vi "Binary_SpectroscopyFile-Open.vi"(8 "error in (no error)":errorcluster, 11 "Binary Spectroscopy File":path) -> (0 "error out":errorcluster, 1 "Config":T1, 2 "Number of Experiments":i32, 3 "File ref":refnum<file>, 5 "Global Attributes":string[][](table))   [LabVIEW 2021, in "Nanonis Prog Interface.lvlib"]
doc: "<b>Opens a binary (.3ds) file and reads the header.</b>\n\nIt will return the file configuration (cluster containing grid resolution, grid position & size, acquired channels etc.) and a file reference.\n\n- Nanonis Programming Interface -"
uses:
  Nanonis Prog Interface.lvlib
  Binary_SpectroscopyFile-Config.ctl
panel:
  out "file size (bytes)":i32
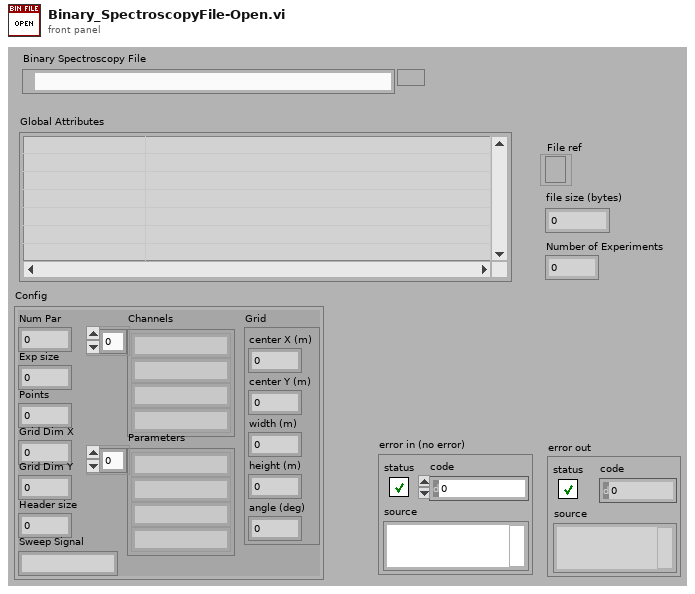
[diagram p1: front panel]
types:
  T1 = typedef "Nanonis Prog Interface.lvlib/Binary_SpectroscopyFile-Config.ctl" = cluster{"Num Par":i32, "Exp size":i32, "Points":i32, "Grid Dim X":i32, "Grid Dim Y":i32, "Header size":i32, "Channels":string[], "Parameters":string[], "Sweep Signal":string, "Grid":cluster{"center X (m)":sgl, "center Y (m)":sgl, "width (m)":sgl, "height (m)":sgl, "angle (deg)":sgl}}
  T2 = cluster{"center X":sgl, "center Y":sgl, "width":sgl, "height":sgl, "angle":sgl}
  T3 = cluster{"[0]":sgl, "[1]":sgl, "[2]":sgl, "[3]":sgl, "[4]":sgl}
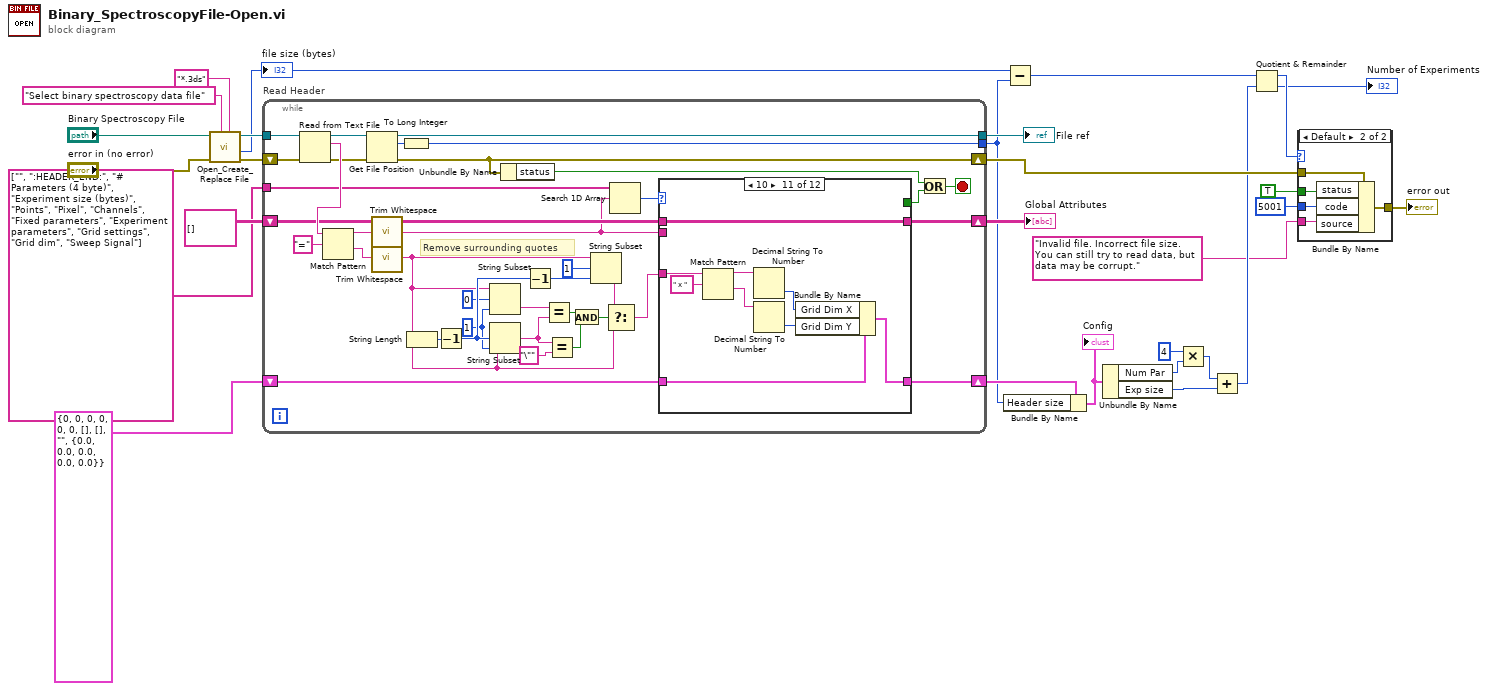
[diagram p0: block diagram]
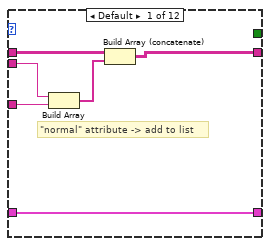
[diagram p3: hidden frame]
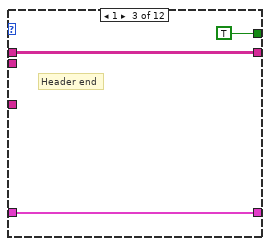
[diagram p5: hidden frame]
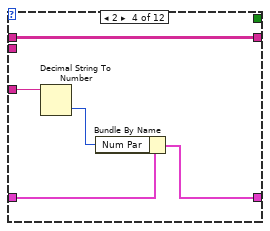
[diagram p6: hidden frame]
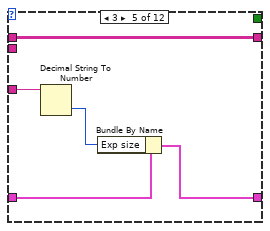
[diagram p7: hidden frame]
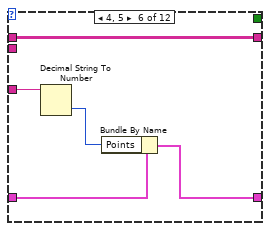
[diagram p8: hidden frame]
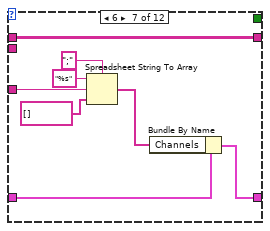
[diagram p9: hidden frame]
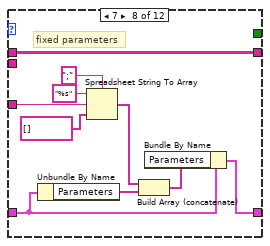
[diagram p10: hidden frame]
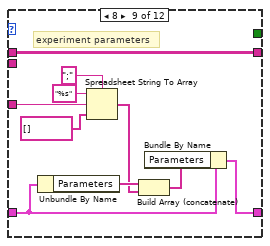
[diagram p11: hidden frame]
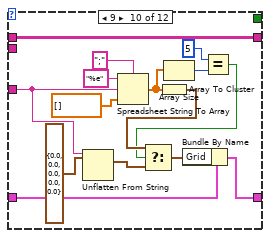
[diagram p12: hidden frame]
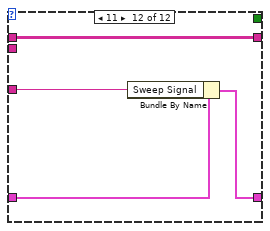
[diagram p13: hidden frame]
diagram:
  n1 = call <vilib>:"Open_Create_Replace File.vi"("pattern"="*.3ds", "prompt"="Select binary spectroscopy data file", "error in (no error)"="error in (no error)", "file path"="Binary Spectroscopy File") -> ("error out"=w25:errorcluster, "file size (bytes)"=w16:i32, "refnum"=w26:refnum<file>)  [unwired: 4 in, 1 out]
  "file size (bytes)" <- w16
  n2 = while "Read Header" {
    tunnel: w26 -> [w65]
    shift-right: [w43] -> w22
    shift-left: string[][] [] -> [w44]
    tunnel: string[] ["", ":HEADER_END:", "# Parameters (4 byte)", "Experiment size (bytes)", "Points", "Pixel", "Channels", "Fixed parameters", "Experiment parameters", "Grid settings", "Grid dim", "Sweep Signal"] -> [w61]
    shift-right: [w41] -> w5
    shift-left: T1 {"Num Par"=0, "Exp size"=0, "Points"=0, "Grid Dim X"=0, "Grid Dim Y"=0, "Header size"=0, "Channels"=[], "Parameters"=[], "Sweep Signal"="", "Grid"={"center X (m)"=0.0, "center Y (m)"=0.0, "width (m)"=0.0, "height (m)"=0.0, "angle (deg)"=0.0}} ("Spectr-BinFile Config") -> [w42]
    tunnel: [w60] -> w15
    shift-right: [w38] -> w14
    shift-left: w25 -> [w64]
    tunnel: [w59] -> w4
    stop <- w36 stop-if-true
    w47 = 1 ("length")
    # "Remove surrounding quotes"
    n3 = Read from Text File(file (use dialog)=w65, error in=w64) -> (refnum out=w31:refnum<file>, text=w63:string, error out=w30:errorcluster)  [unwired: 2 in, 1 out]
    n4 = Match Pattern(string=w63, regular expression="=") -> (before substring=w35:string, after substring=w33:string)  [unwired: 1 in, 2 out]
    n5 = Get File Position(4:w30, 7:w31) -> (0:w38:errorcluster, 2:w29:i64, 3:w60:refnum<file>)
    n6 = call <vilib>:"Trim Whitespace.vi"("string"=w35) -> ("trimmed string"=w34:string)  [unwired: 1 in]
    n7 = call <vilib>:"Trim Whitespace.vi"("string"=w33) -> ("trimmed string"=w32:string)  [unwired: 1 in]
    n8 = To Long Integer(number=w29) -> (32bit integer=w59:i32)
    n9 = String Length(string=w32) -> (length=w49:i32)
    n10 = Decrement(x=w49) -> (x-1=w56:i32)
    n11 = String Subset(string=w32, offset (0)=0, length (rest)=w47) -> (substring=w51:string)
    n12 = String Subset(string=w32, offset (0)=w56, length (rest)=w47) -> (substring=w46:string)
    n13 = Unbundle By Name(w38) -> ("status"=w39:bool)
    n14 = Decrement(x=w56) -> (x-1=w57:i32)
    n15 = Equal?(x=w51, y=w46) -> (x = y?=w52:bool)
    n16 = Equal?(x=w46, y="\"") -> (x = y?=w54:bool)
    n17 = And(x=w52, y=w54) -> (x .and. y?=w50:bool)
    n18 = String Subset(string=w32, offset (0)=1, length (rest)=w57) -> (substring=w58:string)
    n19 = Select(t=w58, s=w50, f=w32) -> (s? t:f=w40:string)
    n20 = Search 1D Array(1D array=w61, element=w34) -> (index of element=w45:i32)  [unwired: 1 in]
    n21 = case shown="10" w45 {
      tunnel: w40 -> [w67 _ _ w79 w84 w89 w96 w107 w117 w124 w140 w144]
      tunnel: w34 -> [w68 _ _ _ _ _ _ _ _ _ _ _]
      tunnel: w44 -> [w71 w73 w76 w81 w86 w91 w99 w109 w119 w134 w143 w147]
      tunnel: [w69 w73 w76 w81 w86 w91 w99 w109 w119 w134 w143 w147] -> w43
      tunnel: w42 -> [w70 w72 w75 w80 w85 w90 w98 w103 w113 w133 w142 w146]
      tunnel: [w70 w72 w75 w77 w82 w87 w97 w108 w118 w132 w141 w145] -> w41
      tunnel: [_ _ TRUE _ _ _ _ _ _ _ _ _] -> w37
      frame Default {
        # "\"normal\" attribute -> add to list"
        n22 = Build Array(w68, w67) -> (w66:string[])
        n23 = Build Array (concatenate)(w71, w66) -> (w69:string[][])
      }
      frame 0 {
        # "No Attribute name => skip"
      }
      frame 1 {
        # "Header end"
      }
      frame 2 {
        n24 = Decimal String To Number(string=w79) -> (number=w78:i32)  [unwired: 2 in, 1 out]
        n25 = Bundle By Name(cluster=w80, "Num Par"=w78) -> (w77:T1)
      }
      frame 3 {
        n26 = Decimal String To Number(string=w84) -> (number=w83:i32)  [unwired: 2 in, 1 out]
        n27 = Bundle By Name(cluster=w85, "Exp size"=w83) -> (w82:T1)
      }
      frame 4, 5 {
        n28 = Decimal String To Number(string=w89) -> (number=w88:i32)  [unwired: 2 in, 1 out]
        n29 = Bundle By Name(cluster=w90, "Points"=w88) -> (w87:T1)
      }
      frame 6 {
        n30 = Spreadsheet String To Array(delimiter (Tab)=";", format string="%s", spreadsheet string=w96, array type (2D Dbl)=string[] []) -> (array=w93:string[])
        n31 = Bundle By Name(cluster=w98, "Channels"=w93) -> (w97:T1)
      }
      frame 7 {
        # "fixed parameters"
        n32 = Unbundle By Name(w103) -> ("Parameters"=w102:string[])
        n33 = Spreadsheet String To Array(delimiter (Tab)=";", format string="%s", spreadsheet string=w107, array type (2D Dbl)=string[] []) -> (array=w101:string[])
        n34 = Build Array (concatenate)(w101, w102) -> (w100:string[])
        n35 = Bundle By Name(cluster=w103, "Parameters"=w100) -> (w108:T1)
      }
      frame 8 {
        # "experiment parameters"
        n36 = Unbundle By Name(w113) -> ("Parameters"=w111:string[])
        n37 = Spreadsheet String To Array(delimiter (Tab)=";", format string="%s", spreadsheet string=w117, array type (2D Dbl)=string[] []) -> (array=w110:string[])
        n38 = Build Array (concatenate)(w111, w110) -> (w112:string[])
        n39 = Bundle By Name(cluster=w113, "Parameters"=w112) -> (w118:T1)
      }
      frame 9 {
        n40 = Unflatten From String(type=T2 {"center X"=0.0, "center Y"=0.0, "width"=0.0, "height"=0.0, "angle"=0.0} ("Grid"), binary string=w124) -> (value=w126:T2)  [unwired: 3 in, 2 out]
        n41 = Spreadsheet String To Array(delimiter (Tab)=";", format string="%e", spreadsheet string=w124, array type (2D Dbl)=sgl[] []) -> (array=w123:sgl[])
        n42 = Array To Cluster(array=w123) -> (cluster=w127:T3)
        n43 = Array Size(array=w123) -> (size(s)=w122:i32)
        n44 = Equal?(x=5, y=w122) -> (x = y?=w120:bool)
        n45 = Select(t=w127, s=w120, f=w126) -> (s? t:f=w125:T2)
        n46 = Bundle By Name(cluster=w133, "Grid"=w125) -> (w132:T1)
      }
      frame 10 {
        n47 = Match Pattern(string=w140, regular expression=" x ") -> (before substring=w138:string, after substring=w137:string)  [unwired: 1 in, 2 out]
        n48 = Decimal String To Number(string=w138) -> (number=w136:i32)  [unwired: 2 in, 1 out]
        n49 = Decimal String To Number(string=w137) -> (number=w135:i32)  [unwired: 2 in, 1 out]
        n50 = Bundle By Name(cluster=w142, "Grid Dim X"=w136, "Grid Dim Y"=w135) -> (w141:T1)
      }
      frame 11 {
        n51 = Bundle By Name(cluster=w146, "Sweep Signal"=w144) -> (w145:T1)
      }
    }
    n52 = Or(x=w39, y=w37) -> (x .or. y?=w36:bool)
  }
  "Global Attributes" <- w22
  "File ref" <- w15
  n53 = Bundle By Name(cluster=w5, "Header size"=w4) -> (w2:T1)
  "Config" <- w2
  n54 = Subtract(x=w16, y=w4) -> (x-y=w11:i32)
  n55 = Unbundle By Name(w2) -> ("Num Par"=w18:i32, "Exp size"=w20:i32)
  n56 = Multiply(x=4, y=w18) -> (x*y=w19:i32)
  n57 = Add(x=w19, y=w20) -> (x+y=w10:i32)
  n58 = Quotient & Remainder(x=w11, y=w10) -> (x-y*floor(x/y)=w9:i32, floor(x/y)=→"Number of Experiments":i32)
  n59 = case shown="Default" w9 {
    tunnel: w14 -> [w148 w153]
    tunnel: [w148 w152] -> w13
    tunnel: 5001 ("code") -> [_ w151]
    tunnel: TRUE ("status") -> [_ w150]
    tunnel: "Invalid file. Incorrect file size. You can still try to read data, but data may be corrupt." ("source") -> [_ w149]
    frame 0 {
    }
    frame Default {
      n60 = Bundle By Name(cluster=w153, "status"=w150, "code"=w151, "source"=w149) -> (w152:errorcluster)
    }
  }
  "error out" <- w13
